vi "NI VeriStand - Read Waveform(s).vi"   [LabVIEW 2020, in "NI_VS Custom Device Waveform API.lvlib"]
doc: "Reads data from a waveform(s) associated with the specified read session."
uses:
  <vilib>/NI VeriStand/Custom Device Waveform API/NI_VS Custom Device Waveform API.lvlib
  <vilib>/NI VeriStand/Custom Device Waveform API/Single Waveform Read (DBL)/Single Waveform Read (DBL).lvclass
  <vilib>/NI VeriStand/Custom Device Waveform API/Single Waveform Read (CDB)/Single Waveform Read (CDB).lvclass
  <vilib>/NI VeriStand/Custom Device Waveform API/Multiple Waveforms Read (CDB)/Multiple Waveforms Read (CDB).lvclass
  <vilib>/NI VeriStand/Custom Device Waveform API/Multiple Waveforms Read (DBL)/Multiple Waveforms Read (DBL).lvclass
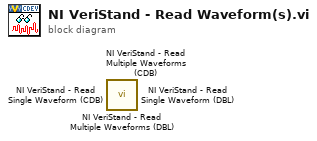
[diagram p0: block diagram]
diagram:
  n1 = call <vilib>:"NI VeriStand - Read Multiple Waveforms (DBL).vi"() -> ()  [unwired: 7 in, 5 out]
  n2 = call <vilib>:"NI VeriStand - Read Multiple Waveforms (CDB).vi"() -> ()  [unwired: 7 in, 5 out]
  n3 = call <vilib>:"NI VeriStand - Read Single Waveform (CDB).vi"() -> ()  [unwired: 7 in, 5 out]
  n4 = call <vilib>:"NI VeriStand - Read Single Waveform (DBL).vi"() -> ()  [unwired: 7 in, 5 out]
